vi "Global.vi"() -> ()   [LabVIEW 2020]
uses:
  <vilib>/_NISVFA/_Shared subVIs/Controls/svc_Spectrum Info.ctl
  <vilib>/_NISVFA/_Shared subVIs/Controls/svc_X-Axis Units.ctl
  <vilib>/_NISVFA/_Shared subVIs/Controls/svc_Spectrum Type.ctl
  <vilib>/_NISVFA/_Shared subVIs/Controls/svc_Engineering Units Text Ring.ctl
  <vilib>/_NISVFA/_Shared subVIs/Controls/svc_Weighting Filter Text Ring.ctl
  <vilib>/_NISVFA/_Shared subVIs/Controls/svc_Complimentary Spectrum Units.ctl
panel:
  out "芯轴码":string
  in  "重试次数":i32
  out "Log":string
  in  "CRC计数":u8
  out "CAN软件版本号":string
  out "K-Line状态":string
  in  "K-Line波特率":u32=38400
  in  "诊断指令":string[][](table)=[["ATI", "MW60K 190630 V3.3"], ["ATSP5", "ISO14230 FastInit"], ["ATSH8131F1", "OK"], ["8100", "7F 81 13"]]
  in  "VISA resource name":refnum<visa-resource-name> caption="COM"
  in  "启用K-line诊断":bool
  out "硬件版本号":string
  out "软件版本号":string
  in  "STOP_NVH":bool
  in  "联机模式":enum16{"单机", "追溯"}(ring)=enum."追溯"
  out "用户信息":T1
  out "产品型号":string
  out "传感器读数":T2 {"吸收电流" format="%#.3f"; "输出扭矩(大)" format="%#.3f"; "输出扭矩(小)" format="%#.3f"; "输入扭矩" format="%#.3f"; "输入编码位移" format="%#.3f"; "工装移载位移" format="%#.3f"; "输入移载位移" format="%#.3f"; "输入旋转位移" format="%#.3f"}
  out "设备状态":i16
  in  "CAN Info":T3={"波特率"=11, "ID"=0, "帧类型"=enum."标准帧", "帧格式"=enum."数据帧", "周期(ms)"=10} {"周期(ms)" min=1 format="%d ms"; "ID" format="0x%x"; "波特率" items=["5Kbps", "10Kbps", "20Kbps", "40Kbps", "50Kbps", "80Kbps", "100Kbps", "125Kbps", "200Kbps", "250Kbps", "400Kbps", "500Kbps", "666Kbps", "800Kbps", "1000Kbps"]}
  in  "输出占空比":refnum<vi>
  out "spectrum info":T4[](array[typedef]) {"x-axis units" items=["Time (s)"=0, "Frequency-CB (Hz)"=1, "Frequency-CPB (Hz)"=1248, "Frequency-Arbitrary (Hz)"=2357, "Quefrency (s)"=2, "Revolutions (rev)"=3, "Order"=4, "Speed (RPM)"=11, "Speed (rad/s)"=21, "Index"=65535]; "weighting filter" items=["Linear", "A-weighting", "B-weighting", "C-weighting", "ITU-R 468-4", "Dolby", "CCITT", "C-message", "Wb", "Wc", "Wd", "We", "Wf", "Wh", "Wj", "Wk", "Wm", "AES17 20 kHz lowpass", "AES17 40 kHz lowpass", "AES17 20 kHz highpass", "AES17 40 kHz highpass"]; "dB reference [EU]" format="%.2f"; "engineering units" items=["custom..."=0, "V"=1, "A"=21, "C"=30, "pC"=31, "s"=32, "-"=29, "Pa"=2, "N"=20, "g"=3, "m/s^2"=4, "m/s"=5, "m"=6, "mm/s"=12, "mm"=13, "micron/s"=14, "micron"=15, "in/s^2"=7, "in/s"=8, "in"=9, "mil/s"=10, "mil"=11, "rad/s^2"=16, "rad/s"=17, "rad"=18, "deg/s^2"=26, "deg/s"=27, "deg"=28, "RPM"=22, "cycle/s^2"=23, "Hz"=24, "cycle"=25, "strain"=19]; "spectral info"."window" items=["None "=0, "Hanning"=1, "Hamming"=2, "Blackman-Harris"=3, "Exact Blackman"=4, "Blackman"=5, "Flat Top"=6, "4 Term B-Harris "=7, "7 Term B-Harris"=8, "Low Sidelobe"=9, "Force - Exponential"=10, "Gaussian"=62]}
  in  "波特率":T10(ring)=enum."500Kbps"
  in  "CAN_CYCLE":T11(array[cluster]) {"周期(ms)" min=1 format="%d ms"; "ID" format="0x%x"}
  in  "启用CAN":bool
  in  "STOP_CAN":bool
  in  "复检判定参数":T12
  out "工位二扭矩偏移":cluster{"正向":dbl, "逆向":dbl}
  out "工位一扭矩偏移":cluster{"正向":dbl, "逆向":dbl}
  out "复检参数":cluster{"复检速度":dbl, "换向扭矩":dbl}
  out "扭矩":cluster{"工位一":dbl, "工位二":dbl}
  out "T2":dbl
  out "T1":dbl
  in  "占空比采集":bool
  out "S7 Link":refnum<k5>
  out "产品编号":string
  in  "计时开始":bool
  in  "计时复位":bool
  in  "IO_Stop":bool
  in  "合格数量":i32
  in  "生产数量":i32
  in  "试验项目":bool[](array[boolean])
  out "模式":u32
  in  "更换产品":refnum<vi>
  in  "提示信息":refnum<vi>
  in  "程序自动":refnum<vi>
  in  "报警图标":refnum<vi>
  in  "程序关闭":bool
  in  "Info":refnum<vi>
  in  "Result":refnum<vi>
  in  "批次":refnum<vi>
  # "帧ID"
  # "帧类型"
  # "帧格式"
  # "帧数据"
  # "周期"
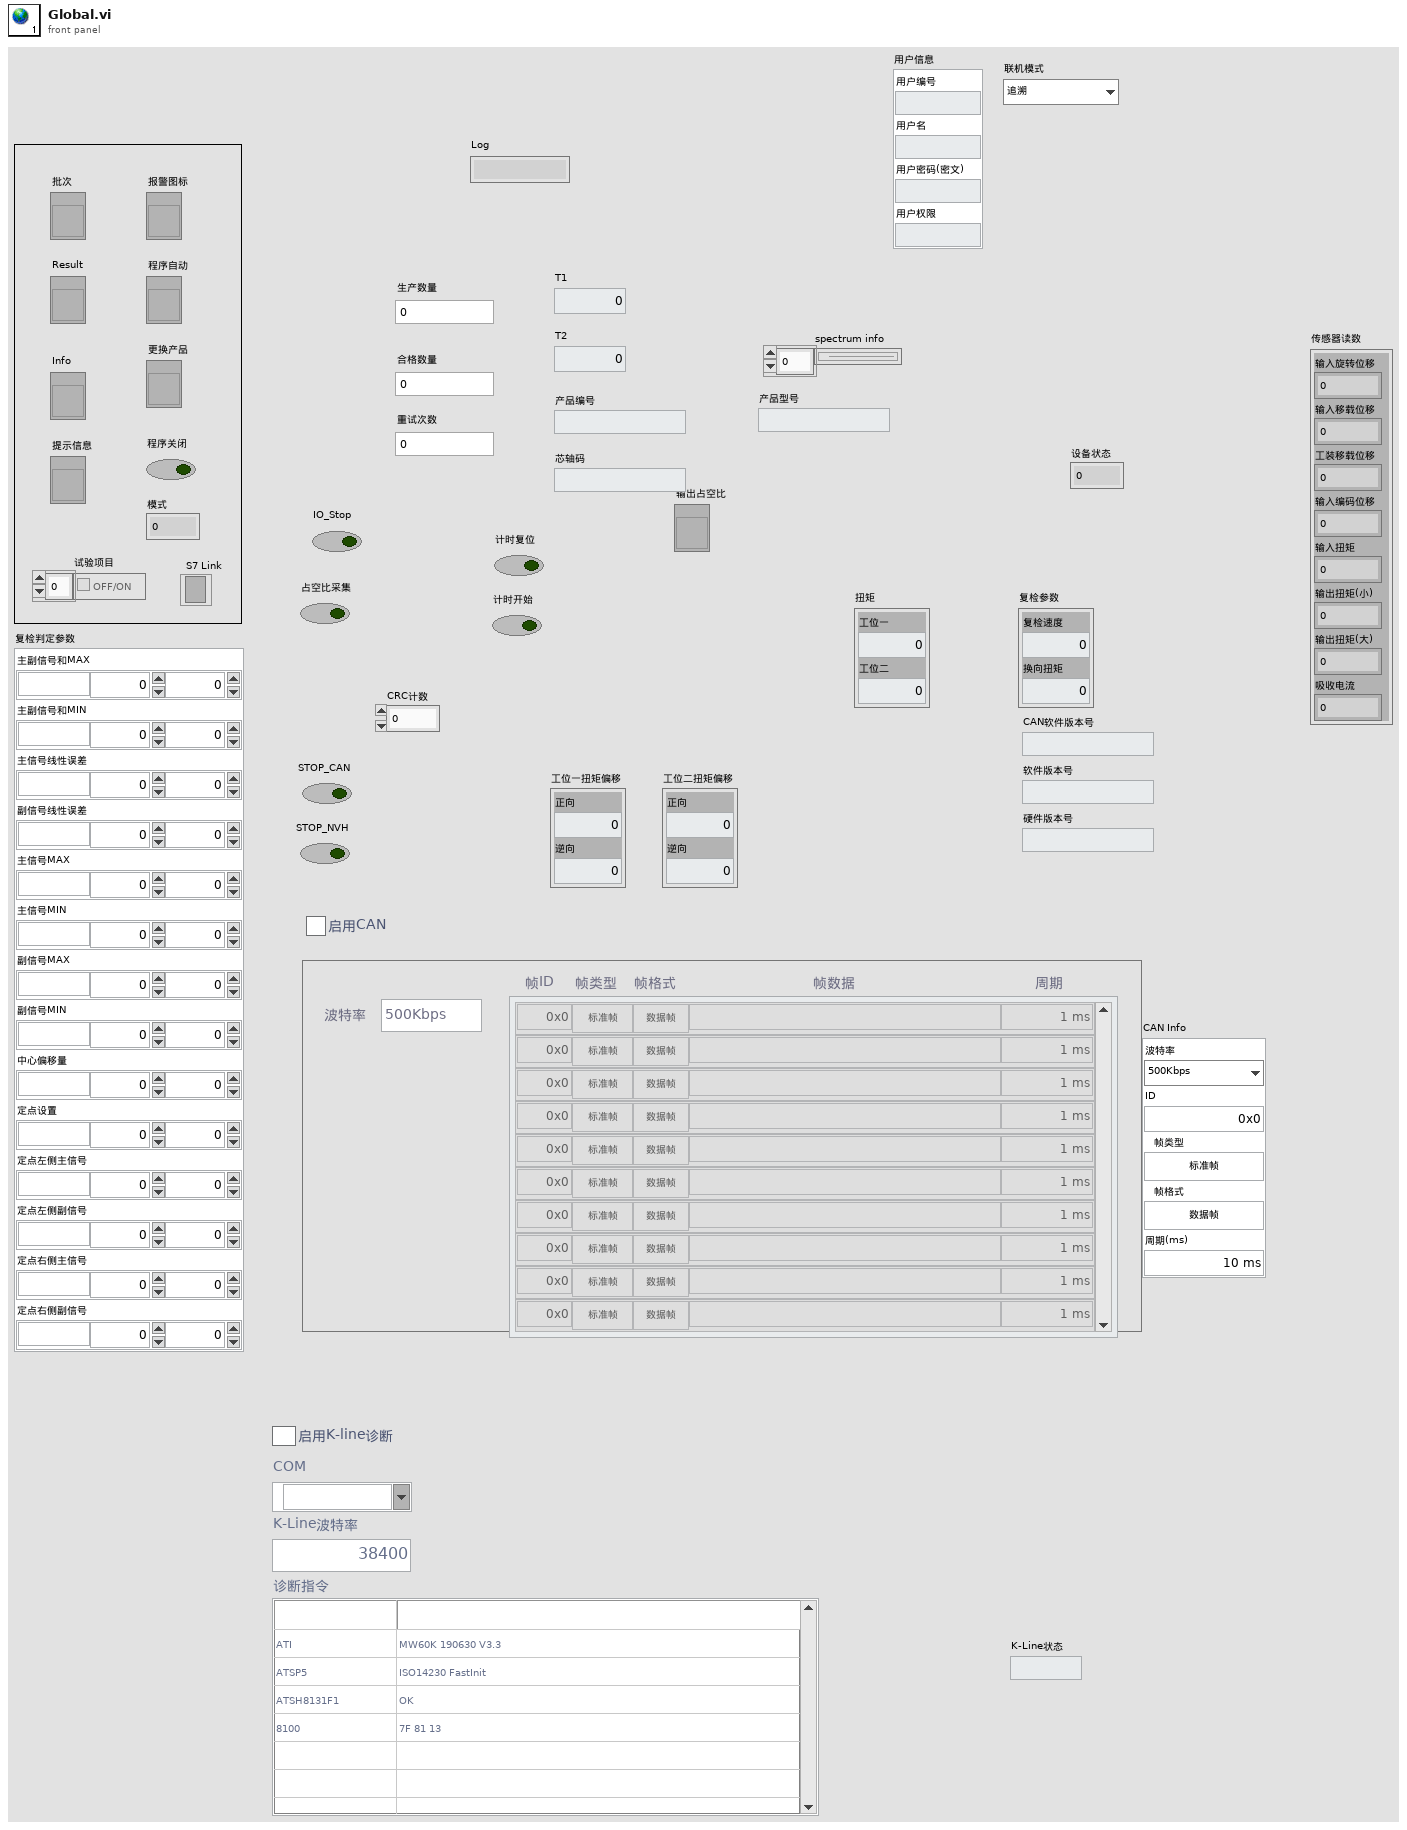
[diagram p1: front panel]
types:
  T1 = cluster{"用户编号":string, "用户名":string, "用户密码(密文)":string, "用户权限":string}
  T2 = cluster{"输入旋转位移":sgl, "输入移载位移":sgl, "工装移载位移":sgl, "输入编码位移":sgl, "输入扭矩":sgl, "输出扭矩(小)":sgl, "输出扭矩(大)":sgl, "吸收电流":sgl}
  T3 = cluster{"波特率":u32, "ID":u32, "帧类型":enum8{"标准帧", "扩展帧"}, "帧格式":enum16{"数据帧", "远程帧"}, "周期(ms)":u32}
  T4 = typedef "svc_Spectrum Info.ctl" = cluster{"channel name":string, "description":string, "x-axis units":T5, "spectral info":cluster{"spectrum type":T6, "linear/dB":enum16{"linear", "dB"}, "window":u16, "window size":i32, "FFT size":i32}, "engineering units":T7, "custom label":string, "dB reference [EU]":dbl, "peak units":enum16{"rms", "peak", "peak-peak"}, "weighting filter":T8, "spectral density?":bool, "unit label":string, "spectrum skewed?":bool, "complimentary spectrum units":T9}
  T5 = typedef "svc_X-Axis Units.ctl" = u16
  T6 = typedef "svc_Spectrum Type.ctl" = enum16{"FFT Spectrum [complex]", "Amplitude [Magnitude]", "Power [Magnitude^2]", "Cross Spectrum [complex]", "Frequency Response [Complex]"}
  T7 = typedef "svc_Engineering Units Text Ring.ctl" = u16
  T8 = typedef "svc_Weighting Filter Text Ring.ctl" = u16
  T9 = typedef "svc_Complimentary Spectrum Units.ctl" = enum16{"none", "radians", "degrees", "cycles", "imaginary"}
  T10 = enum16{"5Kbps", "10Kbps", "20Kbps", "40Kbps", "50Kbps", "80Kbps", "100Kbps", "125Kbps", "200Kbps", "250Kbps", "400Kbps", "500Kbps", "666Kbps", "800Kbps", "1000Kbps"}
  T11 = cluster{"ID":u32, "帧类型":enum8{"标准帧", "扩展帧"}, "帧格式":enum16{"数据帧", "远程帧"}, "帧数据":string, "周期(ms)":u32}[]
  T12 = cluster{"主副信号和MAX":cluster{"单位":string, "下限":dbl, "上限":dbl}, "主副信号和MIN":cluster{"单位":string, "下限":dbl, "上限":dbl}, "主信号线性误差":cluster{"单位":string, "下限":dbl, "上限":dbl}, "副信号线性误差":cluster{"单位":string, "下限":dbl, "上限":dbl}, "主信号MAX":cluster{"单位":string, "下限":dbl, "上限":dbl}, "主信号MIN":cluster{"单位":string, "下限":dbl, "上限":dbl}, "副信号MAX":cluster{"单位":string, "下限":dbl, "上限":dbl}, "副信号MIN":cluster{"单位":string, "下限":dbl, "上限":dbl}, "中心偏移量":cluster{"单位":string, "下限":dbl, "上限":dbl}, "定点设置":cluster{"单位":string, "下限":dbl, "上限":dbl}, "定点左侧主信号":cluster{"单位":string, "下限":dbl, "上限":dbl}, "定点左侧副信号":cluster{"单位":string, "下限":dbl, "上限":dbl}, "定点右侧主信号":cluster{"单位":string, "下限":dbl, "上限":dbl}, "定点右侧副信号":cluster{"单位":string, "下限":dbl, "上限":dbl}}
diagram:
